vi "SP Strip Memory Traces From Waveform.vi"(4 "Sxx Data":waveform(dbl)[](array[waveform])) -> (1 "Sxx Data":waveform(dbl)[](array[waveform]))   [LabVIEW 2011]
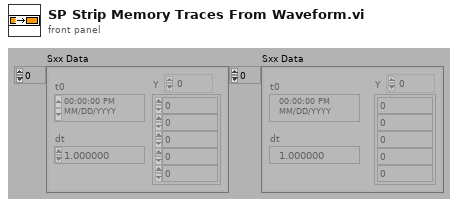
[diagram p1: front panel]
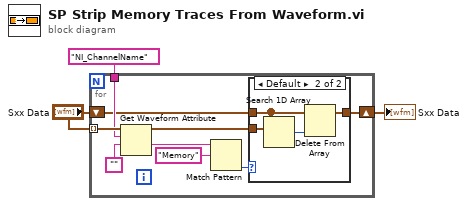
[diagram p0: block diagram]
diagram:
  n1 = for {
    tunnel: "Sxx Data" -> [w12] mode=indexing
    tunnel: "NI_ChannelName" -> [w11]
    shift-right: [w9] -> w3
    shift-left: "Sxx Data" -> [w10]
    n2 = Get Waveform Attribute(5:"", 6:w11, 7:w12) -> (1:w7:string, 3:w4:waveform(dbl))  [unwired: 1 in, 2 out]
    n3 = Match Pattern(string=w7, regular expression="Memory") -> (offset past match=w5:i32)  [unwired: 4 out]
    n4 = case shown="Default" w5 {
      tunnel: w10 -> [w13 w16]
      tunnel: [w13 w17] -> w9
      tunnel: w4 -> [_ w15]
      frame -1 {
      }
      frame Default {
        n5 = Search 1D Array(1D array=w16, element=w15) -> (index of element=w14:i32)  [unwired: 1 out]
        n6 = Delete From Array(array=w16, index=w14) -> (array with subset deleted=w17:waveform(dbl)[])  [unwired: 1 in, 1 out]
      }
    }
  }
  "Sxx Data" <- w3
